vi "CloseCamera.vi"(2 "error in (no error)":errorcluster, 3 "QT Ref In":T1) -> (0 "error out":errorcluster={"status"=TRUE, "code"=-43, "source"=""})   [LabVIEW 2024]
doc: "This VI closes the computer's connection to the camera. It is an important icon that should not be left off. Without closing the connection to the camera, LabVIEW will still think its connection to the camera is open. This may be problematic when you are working on several image processing vi’s or using other applications that require the camera."
uses:
  <userlib>/ImageProcessing/QTLIB_2595_LV86/QT_Ref.ctl
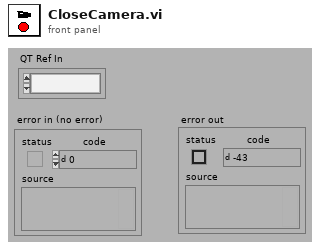
[diagram p1: front panel]
types:
  T1 = typedef "QT_Ref.ctl" = refnum<k1>
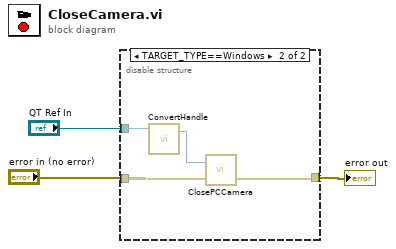
[diagram p0: block diagram]
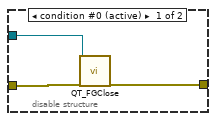
[diagram p2: hidden frame]
diagram:
  n1 = disable-structure shown="TARGET_TYPE==Windows" {
    disable-tunnel: "error in (no error)" -> [w6 w10]
    disable-tunnel: "QT Ref In" -> [w5 w8]
    disable-tunnel: [w4 w9] -> w1
    frame condition #0 (active) {
      n2 = call <userlib>:"QT_FGClose.vi"("QT Ref In"=w5, "error in (no error)"=w6) -> ("error out"=w4:errorcluster)  [unwired: 2 in, 15 out]
    }
    frame condition #1 {
      n3 = call <vilib>:"ConvertHandle.vi"("QT Ref In"=w8) -> ("Camera Reference"=w7:i64)  [unwired: 1 in, 1 out]
      n4 = call <vilib>:"ClosePCCamera.vi"("error in (no error)"=w10, "Camera Reference"=w7) -> ("error out"=w9:errorcluster)  [unwired: 1 in]
    }
  }
  "error out" <- w1
